vi "Sample_multiRecord.vi"() -> ()   [LabVIEW 2013]
doc: "This example demonstrates how to configure multi channels."
uses:
  <userlib>/ArtScope/Trigger/ArtScope_ConfigureTriggerSoftWare.vi
  <userlib>/ArtScope/Fetch/ArtScope_FetchBinary16.vi
  <userlib>/ArtScope/_SubVI/ArtScope_ArrayByChannel_U16.vi
panel:
  in  "band width":i32[](array[ring])=[0, 0] items=["All"=-1, "Default"=0, "100MHz"=1, "20MHz"=2]
  in  "input impendence":i32[](array[ring])=[0, 0] items=["1MΩ", "50Ω"]
  in  "reference position":dbl=100.0
  in  "probe attenuation":i32[](array[numeric])=[1, 1]
  in  "offset(mV)":i32[](array[numeric])=[1000, 5000]
  in  "Stop":bool
  in  "coupling":i32[](array[ring])=[0, 0] items=["DC", "AC"]
  in  "range":i32[](array[ring])=[1, 1] items=["20V", "10V", "2V", "40V", "16V", "8V", "4V", "1.6V", "800m", "400m", "160m", "80m", "40m"]
  in  "channel name":string[](array[string])=["0", "1"]
  out "waveform":u16[][](graph)
  out "error out":errorcluster
  in  "timeout(s)":dbl=10.0
  in  "min record length":i32=1000
  in  "min sample rate":dbl=8000000.0
  in  "resource name":string="Dev1"
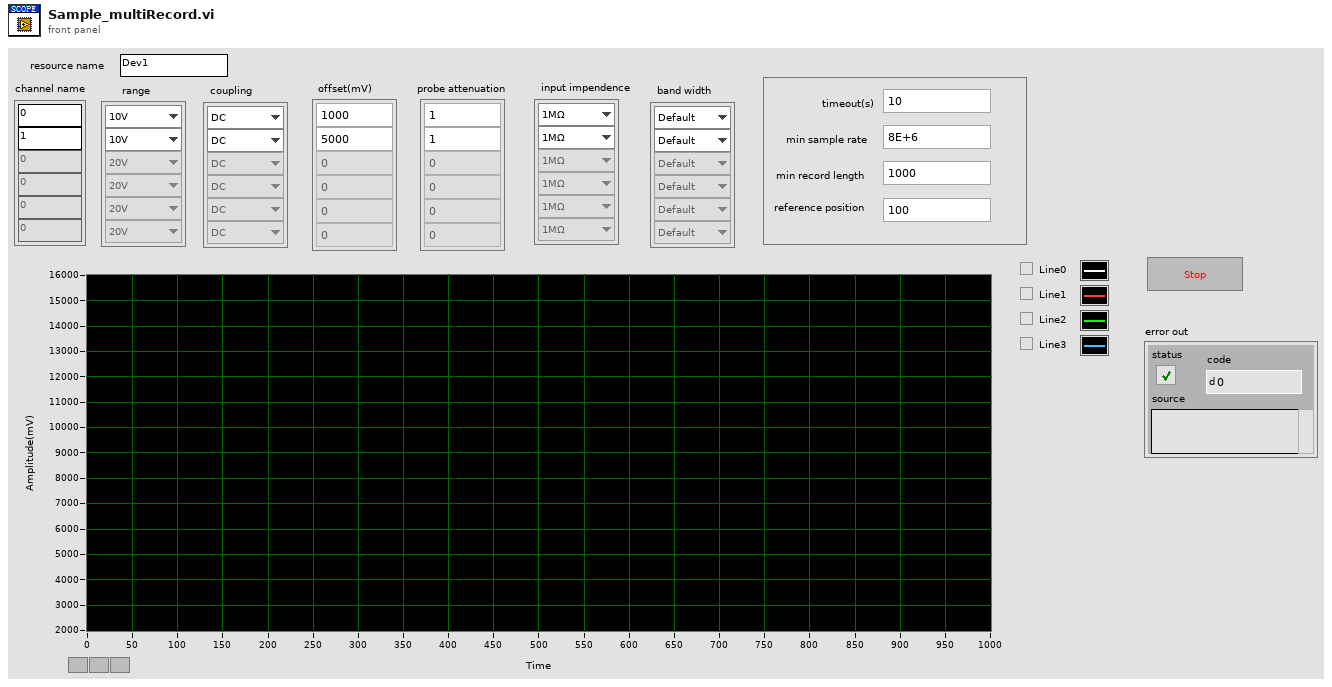
[diagram p1: front panel]
types:
  T1 = cluster{"fLSB":cluster{dbl, dbl, dbl, dbl, dbl, dbl, dbl, dbl}, "RangeValue":cluster{dbl, dbl, dbl, dbl, dbl, dbl, dbl, dbl}, "wMaxLSB":u32, "TriggerMode":i32, "sampLengthPerChan":u32, "pAvailSampsPoints":u32, "channelCount":i32}
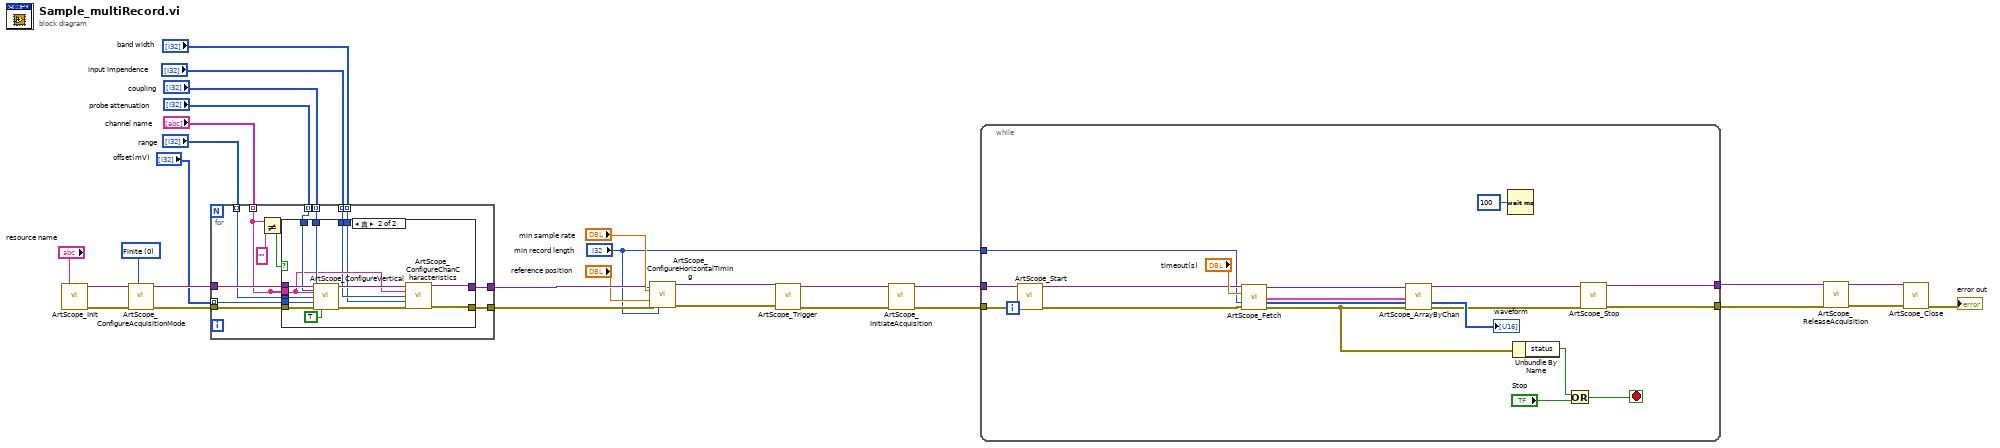
[diagram p0: block diagram]
diagram:
  w23 = 0 items=["Finite", "Continuous"] ("AcuqMode")
  n1 = call <userlib>:"ArtScope_Init.vi"("task name"="resource name") -> ("task handle"=w24:variant, "error out"=w25:errorcluster)  [unwired: 13 in]
  n2 = call <userlib>:"ArtScope_ConfigureAcquisitionMode.vi"("task handle"=w24, "acquisition mode"=w23, "error in (no error)"=w25) -> ("task handle"=w22:variant, "error out"=w26:errorcluster)  [unwired: 11 in]
  n3 = for {
    tunnel: w26 -> [w42]
    tunnel: w22 -> [w41]
    tunnel: [w40] -> w19
    tunnel: [w39] -> w18
    tunnel: "channel name" -> [w32] mode=indexing
    tunnel: "range" -> [w38] mode=indexing
    tunnel: "coupling" -> [w37] mode=indexing
    tunnel: "offset(mV)" -> [w34] mode=indexing
    tunnel: "probe attenuation" -> [w33] mode=indexing
    tunnel: "input impendence" -> [w31] mode=indexing
    tunnel: "band width" -> [w30] mode=indexing
    n4 = Not Equal?(x=w32, y="") -> (x != y?=w36:bool)
    n5 = case shown="真" w36 {
      tunnel: w42 -> [w43 w58]
      tunnel: w41 -> [w44 w57]
      tunnel: [w44 w50] -> w40
      tunnel: [w43 w48] -> w39
      tunnel: w38 -> [_ w56]
      tunnel: w37 -> [_ w55]
      tunnel: w32 -> [_ w47]
      tunnel: w34 -> [_ w54]
      tunnel: w33 -> [_ w52]
      tunnel: w32 -> [_ _]
      tunnel: w31 -> [_ w46]
      tunnel: w30 -> [_ w45]
      frame False {
      }
      frame True {
        n6 = call <userlib>:"ArtScope_ConfigureVertical.vi"("task handle"=w57, "probe attenuation"=w52, "coupling"=w55, "channels"=w47, "range(Vpp)"=w56, "offset"=w54, "error in (no error)"=w58, "enable"=TRUE) -> ("task handle"=w51:variant, "error out"=w49:errorcluster)  [unwired: 6 in]
        n7 = call <userlib>:"ArtScope_ConfigureChanCharacteristics.vi"("task handle"=w51, "channels"=w47, "input impendence"=w46, "bandwidth"=w45, "error in (no error)"=w49) -> ("task handle"=w50:variant, "error out"=w48:errorcluster)  [unwired: 9 in]
      }
    }
  }
  n8 = call <userlib>:"ArtScope_ConfigureHorizontalTiming.vi"("task handle"=w19, "min sample rate"="min sample rate", "reference position"="reference position", "error in (no error)"=w18, "min record length"="min record length") -> ("task handle"=w20:variant, "error out"=w21:errorcluster)  [unwired: 9 in]
  n9 = call-poly <userlib>:"ArtScope_Trigger.vi"("task handle"=w20, "error in (no error)"=w21) -> ("task handle"=w9:variant, "error out"=w8:errorcluster)  [unwired: 12 in]
  n10 = call <userlib>:"ArtScope_InitiateAcquisition.vi"("task handle"=w9, "error in (no error)"=w8) -> ("task handle"=w7:variant, "error out"=w6:errorcluster)  [unwired: 12 in]
  n11 = while {
    tunnel: [w77] -> w10
    tunnel: [w76] -> w13
    tunnel: w7 -> [w72]
    tunnel: w6 -> [w71]
    tunnel: "min record length" -> [w66]
    stop <- w70 stop-if-true
    n12 = call <userlib>:"ArtScope_Start.vi"("task handle"=w72, "error in (no error)"=w71) -> ("task handle"=w68:variant, "error out"=w67:errorcluster)  [unwired: 12 in]
    n13 = call-poly <userlib>:"ArtScope_Fetch.vi"("task handle"=w68, "timeout"="timeout(s)", "num samples"=w66, "error in (no error)"=w67) -> ("task handle"=w64:variant, "wfm info"=w59:T1, "data"=w63:u16[], "error out"=w65:errorcluster)  [unwired: 8 in]
    n14 = call-poly <userlib>:"ArtScope_ArrayByChan.vi"("task handle"=w64, "wfm info"=w59, "1D data"=w63, "error in (no error)"=w65) -> ("task handle"=w61:variant, "2D data"=→"waveform":u16[][], "error out"=w60:errorcluster)  [unwired: 9 in]
    n15 = Wait (ms)(milliseconds to wait=u32 100 ("等待时间（毫秒）")) -> ()  [unwired: 1 out]
    n16 = Unbundle By Name(w65) -> ("status"=w74:bool)
    n17 = Or(x=w74, y="Stop") -> (x .or. y?=w70:bool)
    n18 = call <userlib>:"ArtScope_Stop.vi"("task handle"=w61, "error in (no error)"=w60) -> ("task handle"=w77:variant, "error out"=w76:errorcluster)  [unwired: 12 in]
  }
  n19 = call <userlib>:"ArtScope_ReleaseAcquisition.vi"("task handle"=w10, "error in (no error)"=w13) -> ("task handle"=w11:variant, "error out"=w12:errorcluster)  [unwired: 12 in]
  n20 = call <userlib>:"ArtScope_Close.vi"("task handle"=w11, "error in (no error)"=w12) -> ("error out"=→"error out":errorcluster)  [unwired: 13 in]
